vi "PH_Switch_USB.constructor.vi"(0 "name":string, 2 "data in":string, 5 "error in(no error)":errorcluster) -> (14 "i ref out":refnum<vi>, 16 "data out":string, 19 "error out":errorcluster)   [LabVIEW 2014, in "PH_Switch_USB.lvlib"]
doc: "This class is forseen to control easy switches with up to two end position sensors using Beckhoff.\n\nThis class is part of the PHELIX device layer.\n\nauthor: Stefan Götte, GSI\n\nLicense Agreement for this software:\n\nCopyright (C)\nGesellschaft für Schwerionenforschung, GSI\nPlanckstr. 1\n64291 Darmstadt\nGermany\n\nContact: D.Beck@gsi.de \n\nThis program is free software; you can redistribute it and/or modify it under the terms of the \nGNU General Public License as published by the Free Software Foundation; either version 2 of \nthe license, or (at your option) any later version.\n\nThis program is distributed in the hope that it will be useful, but WITHOUT ANY WARRANTY; \nwithout even the implied warranty of MERCHANTABILITY or FITNESS FOR A PARTICULAR PURPOSE. See the GNU General License for more details (http://www.gnu.org).\n\nGesellschaft für Schwerionenforschung, GSI\nPlanckstr. 1, 64291 Darmstadt, Germany\nFor all questions and ideas contact: M.Richter@gsi.de, H.Brand@gsi.de or D.Beck@gsi.de.\nLast update: 16-JUN-2004"
uses:
  PH_Switch_USB.lvlib
  PH_Basics/PH_Class/PH_Class.lvlib
  PH_Basics/PH_StatusHandler/PH_StatusHandler.lvlib
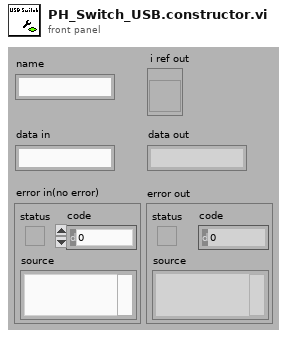
[diagram p1: front panel]
types:
  T1 = enum16{"SetAttribute", "GetAttribute", "CreateAttribute", "DestroyAttribute", "DestroyAllAtributes"}
  T2 = typedef "PH_Switch_USB.lvlib/PH_Switch_USB.i attribute.ctl" = cluster{"GUI Refs":cluster{"GUI-Knob":refnum<vi>, "Delete":refnum<vi>}, "Switch":cluster{"GUI Ref":refnum<vi>, "Service name":string, "Array No.":i16, "caption":string, "Status":T3}, "True-Sensor":cluster{"GUI Ref":refnum<vi>, "Service name":string, "Array No.":i16, "caption":string, "Status":T3}, "False-Sensor":cluster{"GUI Ref":refnum<vi>, "Service name":string, "Array No.":i16, "caption":string, "Status":T3}}
  T3 = typedef "PH_StatusHandler.lvlib/PH_StatusHandler.Status.ctl" = i16
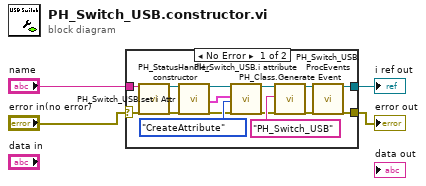
[diagram p0: block diagram]
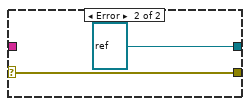
[diagram p2: hidden frame]
diagram:
  n1 = case shown="No Error" "error in(no error)" {
    selector: "error in(no error)" -> [w17 w21]
    tunnel: [w15 refnum<vi> refnum ("i ref out")] -> w4
    tunnel: [w16 w21] -> w3
    tunnel: "name" -> [w19 _]
    frame No Error {
      n2 = call "PH_StatusHandler.constructor.vi"("name"=w19, "error in(no error)"=w17) -> ("i ref out"=w11:refnum<vi>, "error out"=w9:errorcluster)  [unwired: 15 in, 1 out]
      n3 = call "PH_Switch_USB.set i Attr.vi"("i ref in"=w11, "error in (no error)"=w9) -> ("i ref out"=w10:refnum<vi>, "i Attributes"=w7:T2, "error out"=w8:errorcluster)  [unwired: 15 in]
      n4 = call "PH_Switch_USB.i attribute.vi"("VI Refnum"=w10, "CLASS.i attribute"=w7, "Action"=T1."CreateAttribute", "error in (no error)"=w8) -> ("VI Refnum out"=w6:refnum<vi>, "error out"=w5:errorcluster)  [unwired: 13 in, 1 out]
      n5 = call "PH_Class.Generate Event.vi"("i ref in"=w6, "Class"="PH_Switch_USB", "error in (no error)"=w5) -> ("i ref out"=w13:refnum<vi>, "error out"=w14:errorcluster)  [unwired: 15 in]
      n6 = call "PH_Switch_USB.ProcEvents.vi"("i ref in"=w13, "error in (no error)"=w14) -> ("i ref out"=w15:refnum<vi>, "error out"=w16:errorcluster)  [unwired: 16 in]
    }
    frame Error {
    }
  }
  "i ref out" <- w4
  "error out" <- w3
